vi "ComputerNamesReadWrite.vi"() -> ()   [LabVIEW 2022 SP3]
uses:
  -ScanSystem/Controls/location.ctl
  ComputerName.ctl
  <vilib>/Utility/xml.llb/Read From XML File(string).vi
  <vilib>/Utility/xml.llb/Write to XML File(string).vi
panel:
  in  "stop":bool
  in  "Computer Table":cluster{"Computer Name":string, "Location":T1}[](array[cluster])
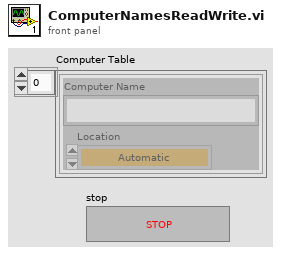
[diagram p1: front panel]
types:
  T1 = typedef "location.ctl" = enum16{"Automatic", "WCM Main", "Hawaii", "Columbia MM3000", "Columbia  NI System", "NYU", "RRI 2", "UHI Allen", "CUMC RT", "Chiba", "Stony Brook", "WCM Microscopy", "WCM Aeoretch", "WCM Optics Lab", "WCM Main 2Axis", "WCM Rotation", "WCM SAM SMAC", "SERI GP"}
  T2 = typedef "ComputerName.ctl" = cluster{"Computer Name":string, "Location":T1}
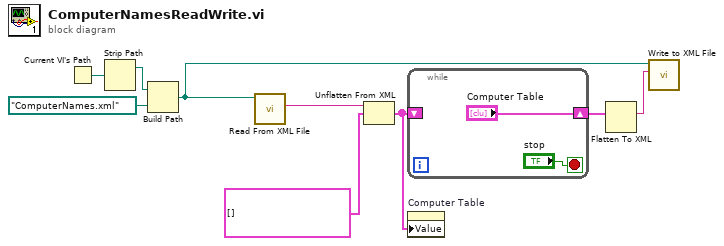
[diagram p0: block diagram]
diagram:
  n1 = Current VI's Path() -> (path=w8:path)
  n2 = Strip Path(path=w8) -> (stripped path=w6:path)  [unwired: 1 out]
  n3 = Build Path(base path=w6, name or relative path=path "ComputerNames.xml" ("path to XML document")) -> (appended path=w1:path)
  n4 = call-poly <vilib>:"Read From XML File.vi"("XML File Path"=w1) -> ("XML Elements"=w9:string)  [unwired: 8 in, 2 out]
  n5 = Unflatten From XML(xml string=w9, type=T2[] []) -> (value=w5:T2[])  [unwired: 1 in, 1 out]
  n6 = while {
    shift-right: ["Computer Table"] -> w2
    shift-left: w5 -> [_]
    stop <- "stop" stop-if-true
  }
  n7 = property on="Computer Table" class="Arr (strict)"("Value"=w5) -> ()  [unwired: 2 in, 2 out]
  n8 = Flatten To XML(6:w2) -> (2:w3:string)
  n9 = call-poly <vilib>:"Write to XML File.vi"("XML Input"=w3, "XML File Path"=w1) -> ()  [unwired: 7 in, 3 out]
